vi "报警定义配置.vi"() -> ()   [LabVIEW 2016, in "Alarm interface.lvlib"]
uses:
  Alarm interface.lvlib
  <vilib>/Utility/miscctls.llb/LVPointTypeDef.ctl
panel:
  in  "关闭":bool
  in  "三级报警":string[][](table)
  in  "二级报警":string[][](table)
  in  "报警定义表":i32(listbox)
  in  "一级报警":string[][](table)
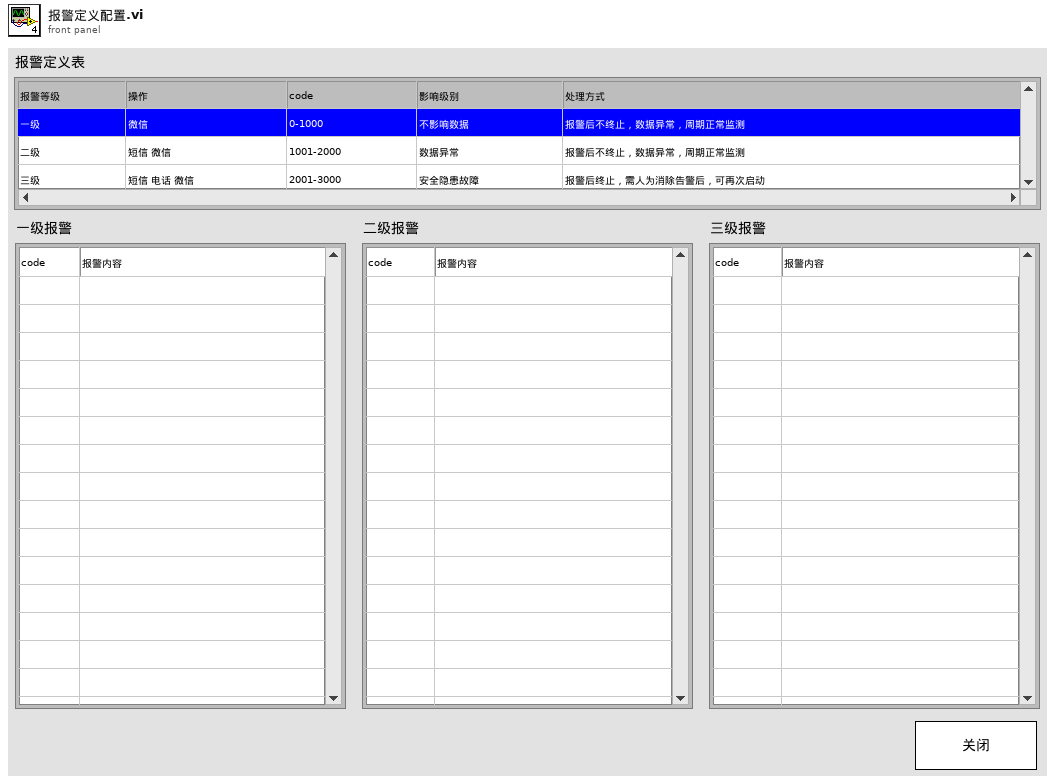
[diagram p1: front panel]
types:
  T1 = typedef "LVPointTypeDef.ctl" = cluster{"Horizontal":i16, "Vertical":i16}
  T2 = cluster{"一级告警":string[][], "二级告警":string[][], "三级告警":string[][]}
  T3 = typedef "LVPoint32TypeDef.ctl" = cluster{"Horizontal":i32, "Vertical":i32}
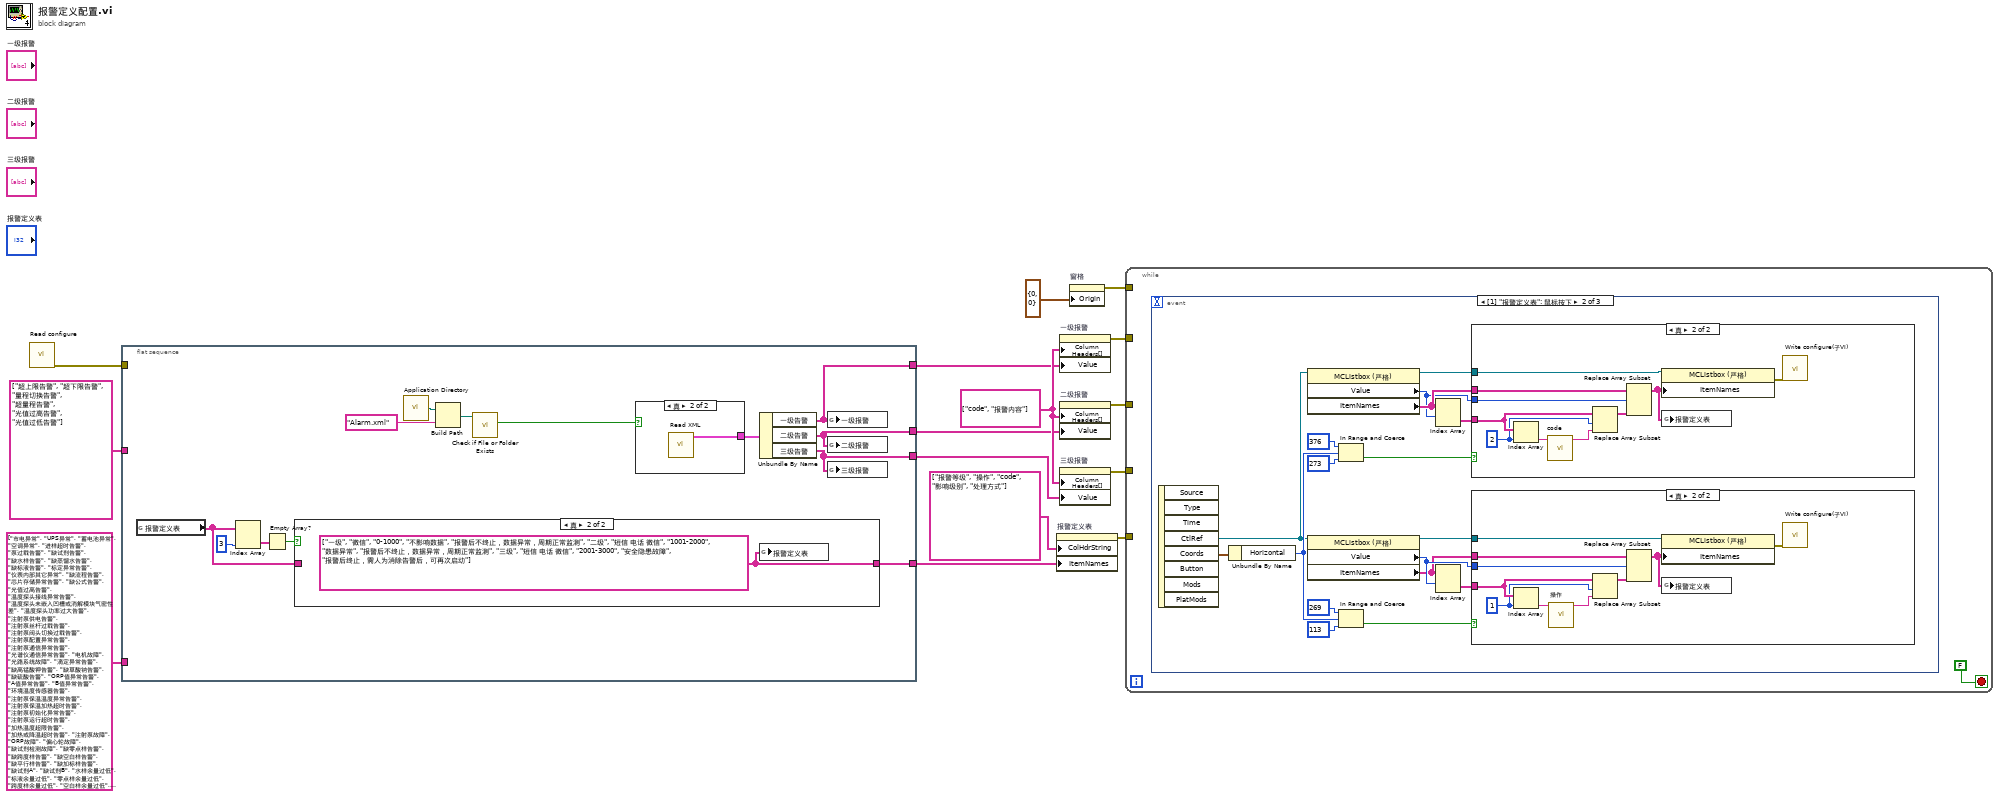
[diagram p0: block diagram]
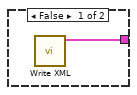
[diagram p2: hidden frame]
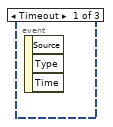
[diagram p4: hidden frame]
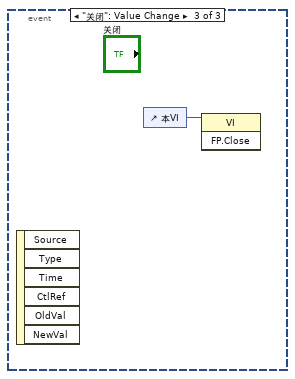
[diagram p7: hidden frame]
diagram:
  w11 = string[] ["code", "报警内容"] ("列首字符串[]")
  n1 = call "Read configure.vi"() -> ("error out"=w12:errorcluster)  [unwired: 11 in]
  n2 = flat-sequence {
    tunnel: w12 -> [_]
    tunnel: [w27] -> w13
    tunnel: [w16] -> w1
    tunnel: [w18] -> w2
    tunnel: [w17] -> w5
    tunnel: string[] ["超上限告警", "超下限告警", "量程切换告警", "超量程告警", "光值过高告警", "光值过低告警"] ("转置的数组") -> [_]
    tunnel: string[] ["市电异常", "UPS异常", "蓄电池异常", "空调异常", "进样超时告警", "泵过载告警", "缺试剂告警", "缺水样告警", "缺蒸馏水告警", "缺标液告警", "标定异常告警", "仪表内部其它异常", "缺流程告警", "芯片存储异常告警", "缺公式告警", "光值过高告警", "温度探头接线异常告警", "温度探头未嵌入凹槽或消解模块气密性差", "温度探头功率过大告警", "注射泵供电告警", "注射泵丝杆过载告警", "注射泵阀头切换过载告警", "注射泵配置异常告警", "注射泵通信异常告警", "光谱仪通信异常告警", "电机故障", "光路系统故障", "滴定异常告警", "缺高锰酸钾告警", "缺草酸钠告警", "缺硫酸告警", "ORP值异常告警", "A值异常告警", "B值异常告警", "环境温度传感器告警", "注射泵保温温度异常告警", "注射泵保温加热超时告警", "注射泵初始化异常告警", "注射泵运行超时告警", "加热温度超限告警", "加热或降温超时告警", "注射泵故障", "ORP故障", "偏心轮故障", "缺试剂检测故障", "缺零点样告警", "缺跨度样告警", "缺空白样告警", "缺平行样告警", "缺加标样告警", "缺试剂A", "缺试剂B", "水样余量过低", "标液余量过低", "零点样余量过低", "跨度样余量过低", "空白样余量过低", "平行样余量过低", "加标样余量过低", "试剂A余量过低", "试剂B余量过低", "请注意查看溶液或试剂余量并及时维护", "旋转阀通信异常告警", "旋转阀故障", "光路系统故障", "液位异常告警", "柱塞泵故障告警", "流程中断告警"] ("转置的数组") -> [_]
    frame #0 {
      n3 = global read "断电保存全局.vi" "报警定义表"() -> (w26:string[][])
      n4 = Index Array(array=w26, index (col)=3 ("禁用的索引 (列)")) -> (element=w24:string[])  [unwired: 1 in]
      n5 = Empty Array?(array=w24) -> (empty?=w28:bool)
      n6 = case shown="真" w28 {
        tunnel: w26 -> [w31 _]
        tunnel: [w31 w32] -> w27
        frame False {
        }
        frame True {
          w32 = string[][] [["一级", "微信", "0-1000", "不影响数据", "报警后不终止，数据异常，周期正常监测"], ["二级", "短信 电话 微信", "1001-2000", "数据异常", "报警后不终止，数据异常，周期正常监测"], ["三级", "短信 电话 微信", "2001-3000", "安全隐患故障", "报警后终止，需人为消除告警后，可再次启动"]] ("报警定义表")
          n7 = global write "断电保存全局.vi" "报警定义表"(w32) -> ()
        }
      }
      n8 = call <vilib>:"Application Directory.vi"() -> ("Application Directory"=w23:path)
      n9 = Build Path(base path=w23, name or relative path="Alarm.xml" ("名称或相对路径")) -> (appended path=w21:path)
      n10 = call <vilib>:"Check if File or Folder Exists.vi"("path"=w21) -> ("file or folder exists?"=w20:bool)  [unwired: 8 in, 2 out]
      n11 = case shown="真" w20 {
        tunnel: [w29 w30] -> w19
        frame False {
          n12 = call "Write XML.vi"() -> ("值"=w29:T2)  [unwired: 10 in, 1 out]
        }
        frame True {
          n13 = call "Read XML.vi"() -> ("值"=w30:T2)  [unwired: 10 in, 1 out]
        }
      }
      n14 = Unbundle By Name(w19) -> ("一级告警"=w16:string[][], "二级告警"=w18:string[][], "三级告警"=w17:string[][])
      n15 = global write "断电保存全局.vi" "一级报警"(w16) -> ()
      n16 = global write "断电保存全局.vi" "二级报警"(w18) -> ()
      n17 = global write "断电保存全局.vi" "三级报警"(w17) -> ()
    }
  }
  n18 = property on="报警定义表" class="MCListbox (严格)"("ColHdrString"=string[] ["报警等级", "操作", "code", "影响级别", "处理方式"] ("列首字符串[]"), "ItemNames"=w13) -> (error out=w14:errorcluster)  [unwired: 2 in, 1 out]
  n19 = property on="一级报警" class="Tbl (严格)"("Column Headers[]"=w11, "Value"=w1) -> (error out=w10:errorcluster)  [unwired: 2 in, 1 out]
  n20 = property on="二级报警" class="Tbl (严格)"("Column Headers[]"=w11, "Value"=w2) -> (error out=w9:errorcluster)  [unwired: 2 in, 1 out]
  n21 = property on="三级报警" class="Tbl (严格)"("Column Headers[]"=w11, "Value"=w5) -> (error out=w8:errorcluster)  [unwired: 2 in, 1 out]
  n22 = property on="窗格" class="Pane"("Origin"=T1 {"Horizontal"=0, "Vertical"=0} ("原点")) -> (error out=w6:errorcluster)  [unwired: 2 in, 1 out]
  n23 = while {
    tunnel: w14 -> [_]
    tunnel: w10 -> [_]
    tunnel: w9 -> [_]
    tunnel: w8 -> [_]
    tunnel: w6 -> [_]
    stop <- FALSE stop-if-true
    n24 = event shown="[1] \"报警定义表\": 鼠标按下" {
      selector: _ -> [_ _ _]
      dyn-events: _ -> [_ _ _]
      timeout: _ -> [_ _ _]
      event Timeout {
        n25 = event-data() -> ()  [unwired: 1 in, 3 out]
      }
      event "报警定义表": Mouse Down {
        n26 = event-data() -> ("CtlRef"=w34:refnum<vi>, "Coords"=w50:T3)  [unwired: 1 in, 6 out]
        n27 = Unbundle By Name(w50) -> ("Horizontal"=w49:i32)
        n28 = property class="MCListbox (严格)"(reference=w34) -> (reference out=w42:refnum<vi>, "Value"=w40:i32, "ItemNames"=w41:string[][])  [unwired: 1 in, 1 out]
        n29 = property class="MCListbox (严格)"(reference=w34) -> (reference out=w37:refnum<vi>, "Value"=w39:i32, "ItemNames"=w38:string[][])  [unwired: 1 in, 1 out]
        n30 = In Range and Coerce(upper limit=376 ("下限"), x=w49, lower limit=273 ("上限")) -> (In Range?=w44:bool)  [unwired: 1 out]
        n31 = In Range and Coerce(upper limit=269 ("下限"), x=w49, lower limit=113 ("上限")) -> (In Range?=w35:bool)  [unwired: 1 out]
        n32 = Index Array(array=w41, index (row)=w40) -> (element=w43:string[])  [unwired: 1 in]
        n33 = Index Array(array=w38, index (row)=w39) -> (element=w36:string[])  [unwired: 1 in]
        n34 = case shown="真" w44 {
          tunnel: w43 -> [_ w69]
          tunnel: w42 -> [_ w67]
          tunnel: w41 -> [_ w66]
          tunnel: w40 -> [_ w65]
          frame False {
          }
          frame True {
            w63 = 2 ("索引")
            n35 = Index Array(array=w69, index=w63) -> (element=w70:string)
            n36 = call "code.vi"("字符串输入"=w70) -> ("字符串输出"=w68:string)  [unwired: 10 in]
            n37 = Replace Array Subset(array=w69, new element=w68, index=w63) -> (w64:string[])
            n38 = Replace Array Subset(array=w66, new element=w64, index (row)=w65) -> (w62:string[][])  [unwired: 1 in]
            n39 = property class="MCListbox (严格)"(reference=w67, "ItemNames"=w62) -> (error out=w61:errorcluster)  [unwired: 1 in, 1 out]
            n40 = global write "断电保存全局.vi" "报警定义表"(w62) -> ()
            n41 = call "Write configure(子VI).vi"("error in (no error)"=w61) -> ()  [unwired: 10 in, 1 out]
          }
        }
        n42 = case shown="真" w35 {
          tunnel: w36 -> [_ w60]
          tunnel: w37 -> [_ w59]
          tunnel: w38 -> [_ w58]
          tunnel: w39 -> [_ w57]
          frame False {
          }
          frame True {
            w55 = 1 ("索引")
            n43 = Index Array(array=w60, index=w55) -> (element=w54:string)
            n44 = call "操作.vi"("字符串输入"=w54) -> ("字符串输出"=w53:string)  [unwired: 10 in]
            n45 = Replace Array Subset(array=w60, new element=w53, index=w55) -> (w56:string[])
            n46 = Replace Array Subset(array=w58, new element=w56, index (row)=w57) -> (w52:string[][])  [unwired: 1 in]
            n47 = property class="MCListbox (严格)"(reference=w59, "ItemNames"=w52) -> (error out=w51:errorcluster)  [unwired: 1 in, 1 out]
            n48 = global write "断电保存全局.vi" "报警定义表"(w52) -> ()
            n49 = call "Write configure(子VI).vi"("error in (no error)"=w51) -> ()  [unwired: 10 in, 1 out]
          }
        }
      }
      event "关闭": Value Change {
        n50 = event-data() -> ()  [unwired: 1 in, 6 out]
        n51 = control-ref of="本VI"() -> (w71:refnum<vi>)
        n52 = invoke class="VI" method="FP.Close"(reference=w71) -> ()  [unwired: 2 in, 3 out]
      }
    }
  }
